vi "Qrcode scanner.vi"() -> ()   [LabVIEW 2019]
uses:
  <vilib>/userDefined/High Color/IMAQdx.ctl
  <vilib>/vision/driver/NI_Vision_Acquisition_Software.lvlib
  <vilib>/vision/NI_Vision_Development_Module.lvlib
panel:
  out "Array":string[](array[string])
  out "Data":string
  out "Image":T1(plugin-control)
  out "Found?":bool
  in  "Session In":T2
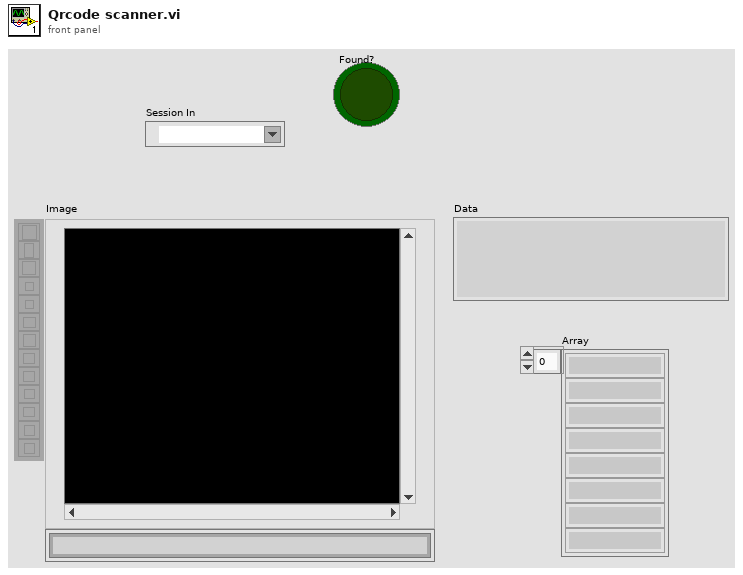
[diagram p1: front panel]
types:
  T1 = typedef "IMAQ Image.ctl" = refnum<image>
  T2 = typedef "IMAQdx.ctl" = refnum<k21>
  T3 = typedef "Image Type" = u32
  T4 = typedef "QR Code Report.ctl" = cluster{"Found?":bool, "Data":string, "Bounding Box":cluster{"x":sgl, "y":sgl}[], "Errors Corrected":u32, "Dimensions (Rows/Cols)":u32, "Version":u32, "QR Model":T5, "Stream Mode":T6, "Barcode Polarity":T7, "Mirrored?":bool, "Append Stream Position":u32, "Size of Append Stream":u32, "First EAN-128 ID":i32, "First Alternate Language ID":i32, "Append Stream ID":u32, "Minimum Edge Strength":u32, "Demodulation Mode":T8, "Cell Sample Size":T9, "Cell Filter Mode":T10}
  T5 = typedef "QR Code Model Type.ctl" = i32
  T6 = typedef "QR Code Stream Mode Type.ctl" = i32
  T7 = typedef "Data Matrix Polarity.ctl" = i32
  T8 = typedef "Demodulation Mode.ctl" = i32
  T9 = typedef "Cell Sample Size.ctl" = i32
  T10 = typedef "Cell Filter Mode.ctl" = i32
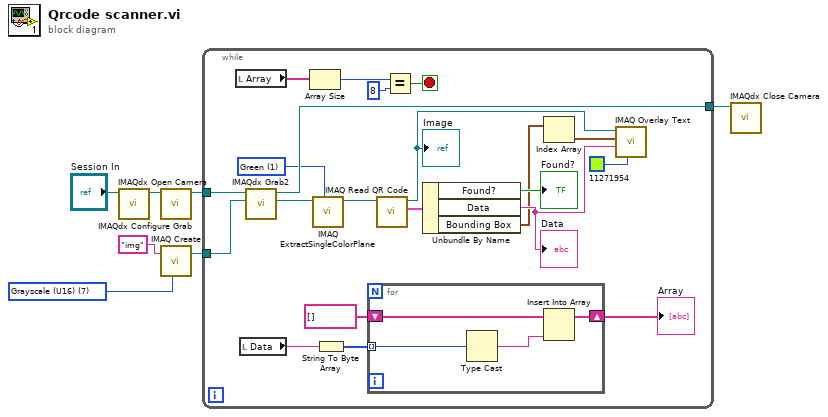
[diagram p0: block diagram]
diagram:
  w2 = T3 7 items=["Grayscale (U8)", "Grayscale (I16)", "Grayscale (SGL)", "Complex (CSG)", "RGB (U32)", "HSL (U32)", "RGB (U64)", "Grayscale (U16)"] ("Image Type")
  n1 = call <vilib>:"IMAQdx Open Camera.vi"("Session In"="Session In") -> ("Session Out"=w6:T2)  [unwired: 9 in, 1 out]
  n2 = call <vilib>:"IMAQdx Configure Grab.vi"("Session In"=w6) -> ("Session Out"=w4:T2)  [unwired: 9 in, 1 out]
  n3 = call "IMAQ Create"("Image Name"="img", "Image Type"=w2) -> ("New Image"=w1:T1)  [unwired: 3 in, 1 out]
  n4 = while {
    tunnel: [w28] -> w5
    tunnel: w4 -> [w27]
    tunnel: w1 -> [w26]
    stop <- w11 stop-if-true
    w23 = 1 items=["Red", "Green", "Blue", "Hue", "Saturation", "Luminance", "Value", "Intensity"] ("Color Plane")
    n5 = local read "Array"() -> (w10:string[])
    n6 = local read "Data"() -> (w12:string)
    n7 = call <vilib>:"IMAQdx Grab2.vi"("Image In"=w26, "Session In"=w27) -> ("Image Out"=w25:T1, "Session Out"=w28:T2)  [unwired: 6 in, 2 out]
    n8 = Array Size(array=w10) -> (size(s)=w9:i32)
    n9 = call "IMAQ ExtractSingleColorPlane"("Color Plane"=w23, "Image Src"=w25) -> ("Image Dst Out"=w24:T1)  [unwired: 8 in, 1 out]
    n10 = String To Byte Array(string=w12) -> (unsigned byte array=w15:u8[])
    n11 = for {
      tunnel: w15 -> [w32] mode=indexing
      shift-right: [w29] -> w13
      shift-left: string[] [] -> [w31]
      n12 = Type Cast(x=w32) -> (*(type *) &x=w30:string)  [unwired: 1 in]
      n13 = Insert Into Array(array=w31, new element=w30) -> (w29:string[])  [unwired: 1 in]
    }
    "Array" <- w13
    n14 = call "IMAQ Read QR Code"("Image"=w24) -> ("QR Code Report"=w22:T4, "Image (duplicate)"=w16:T1)  [unwired: 7 in, 2 out]
    "Image" <- w16
    n15 = Equal?(x=w9, y=8) -> (x = y?=w11:bool)
    n16 = Unbundle By Name(w22) -> ("Found?"=→"Found?":bool, "Data"=w19:string, "Bounding Box"=w17:cluster{"x":sgl, "y":sgl}[])
    "Data" <- w19
    n17 = Index Array(array=w17) -> (element=w20:cluster{"x":sgl, "y":sgl})  [unwired: 1 in]
    n18 = call "IMAQ Overlay Text"("Text Color (black)"=u32 11271954, "String"=w19, "Origin"=w20, "Image"=w16) -> ()  [unwired: 6 in, 2 out]
  }
  n19 = call <vilib>:"IMAQdx Close Camera.vi"("Session In"=w5) -> ()  [unwired: 10 in, 1 out]
